vi "LED Display Lookup.vi"(1 "Input":u8) -> (0 "Output":u8)   [LabVIEW 2015]
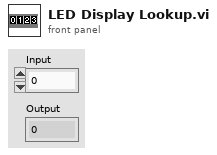
[diagram p1: front panel]
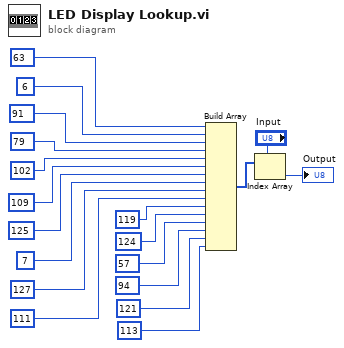
[diagram p0: block diagram]
diagram:
  n1 = Build Array(u8 63, u8 6, u8 91, u8 79, u8 102, u8 109, u8 125, u8 7, u8 127, u8 111, u8 119, u8 124, u8 57, u8 94, u8 121, u8 113) -> (w17:u8[])
  n2 = Index Array(array=w17, index="Input") -> (element=→"Output":u8)
